vi "Simple Range Generator.vi"(4 "Max (T) / Step (F)":bool=TRUE, 5 "Max/Step":dbl, 6 "Min":dbl, 7 "Size":dbl) -> (0 "Min Range":dbl, 1 "Max Range":dbl, 2 "Step Size":dbl, 3 "Array":dbl[](array[numeric]))   [LabVIEW 2017]
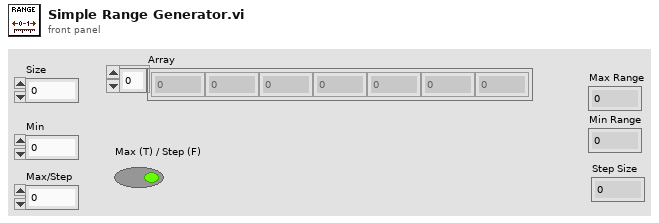
[diagram p1: front panel]
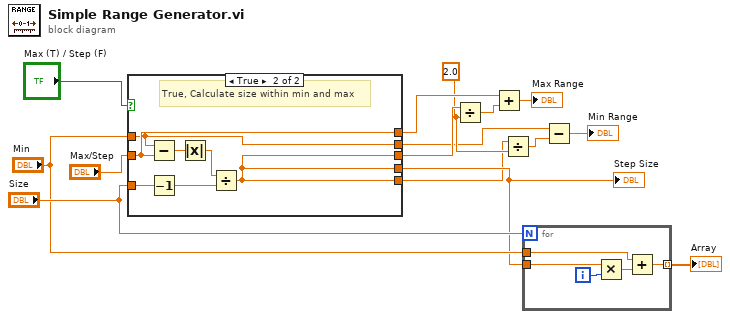
[diagram p0: block diagram]
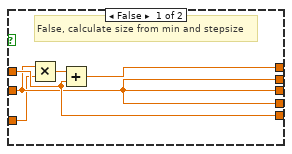
[diagram p2: hidden frame]
diagram:
  w3 = 2.0 ("y")
  n1 = case shown="True" "Max (T) / Step (F)" {
    tunnel: "Size" -> [w17 w24]
    tunnel: "Max/Step" -> [w18 w23]
    tunnel: "Min" -> [w20 w21]
    tunnel: [w18 w22] -> w11
    tunnel: [w18 w22] -> w8
    tunnel: [w16 w23] -> w7
    tunnel: [w20 w22] -> w1
    tunnel: [w18 w21] -> w2
    frame False {
      # "False, calculate size from min and stepsize"
      n2 = Multiply(x=w18, y=w17) -> (x*y=w19:dbl)
      n3 = Add(x=w19, y=w20) -> (x+y=w16:dbl)
    }
    frame True {
      # "True, Calculate size within min and max"
      n4 = Subtract(x=w21, y=w23) -> (x-y=w27:dbl)
      n5 = Decrement(x=w24) -> (x-1=w25:dbl)
      n6 = Absolute Value(x=w27) -> (abs(x)=w26:dbl)
      n7 = Divide(x=w26, y=w25) -> (x/y=w22:dbl)
    }
  }
  "Step Size" <- w11
  n8 = Divide(x=w8, y=w3) -> (x/y=w9:dbl)
  n9 = Add(x=w7, y=w9) -> (x+y=→"Max Range":dbl)
  n10 = Divide(x=w1, y=w3) -> (x/y=w5:dbl)
  n11 = for {
    N: "Size" -> [_]
    tunnel: w11 -> [w32]
    tunnel: "Min" -> [w29]
    tunnel: [w28] -> w15 mode=indexing
    i -> [w31]
    n12 = Multiply(x=w32, y=w31) -> (x*y=w30:dbl)
    n13 = Add(x=w29, y=w30) -> (x+y=w28:dbl)
  }
  "Array" <- w15
  n14 = Subtract(x=w2, y=w5) -> (x-y=→"Min Range":dbl)
